vi "simx Auxiliary Console Print.vi"(7 "operationMode":i32, 8 "error in (no error)":errorcluster, 9 "txt":string, 10 "consoleHandle":i32, 11 "clientID":i32) -> (0 "error out":errorcluster, 3 "function return":i32)   [LabVIEW 2019, in "PXL_V-REP.lvlib"]
doc: "EXTAPI_DLLEXPORT simxInt simxAuxiliaryConsolePrint(simxInt clientID,simxInt consoleHandle,const simxChar* txt,simxInt operationMode);"
uses:
  PXL_V-REP.lvlib
  <userlib>/V-REP/remoteApi.dll
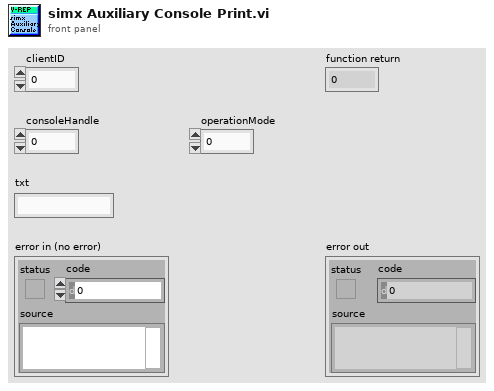
[diagram p1: front panel]
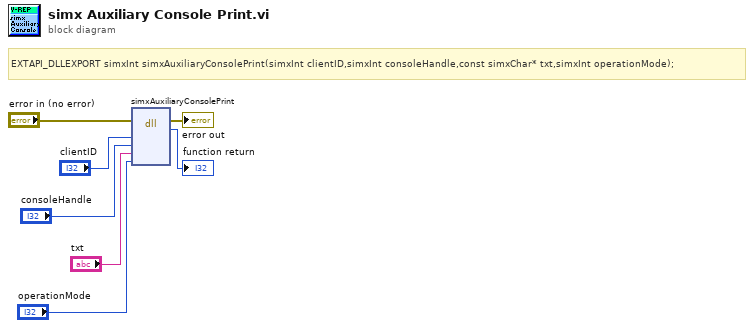
[diagram p0: block diagram]
diagram:
  # "EXTAPI_DLLEXPORT simxInt simxAuxiliaryConsolePrint(simxInt clientID,simxInt consoleHandle,const simxChar* txt,simxInt operationMode);"
  n1 = dll-call lib="C:/Program Files (x86)/National Instruments/LabVIEW 2019/user.lib/V-REP/remoteApi.*" fn="simxAuxiliaryConsolePrint"(error in="error in (no error)", "clientID"="clientID", "consoleHandle"="consoleHandle", "txt"="txt", "operationMode"="operationMode") -> (error out=→"error out":errorcluster, →"function return":i32)  [unwired: 6 in, 1 out]
